vi "final_usrp_transceiver_webcam.vi"() -> ()   [LabVIEW 2014]
uses:
  <vilib>/userdefined/High Color/IMAQdx.ctl
  <vilib>/addons/Modulation/Analog/support/mod_Set Error Source.vi
  var_stop.vi
  <vilib>/addons/Modulation/Digital/Support/Common/Validators/mod_Generate Filter Coefficients Validate.vi
  <vilib>/addons/Modulation/Digital/General/subVIs/mod_Generate Filter Coefficients.vi
  <vilib>/measure/maspectr.llb/FFT Power Spectrum and PSD for 1 Chan (CDB).vi
  <vilib>/addons/Modulation/Digital/General/MT Apply Matched Filter (Generic).vi
  <vilib>/addons/Modulation/Digital/General/MT Align to Ideal Symbols (Generic).vi
  <instrlib>/niUSRP/niUSRP Fetch Rx Data (CDB Cluster).vi
  <instrlib>/niUSRP/niUSRP Write Tx Data (CDB Cluster).vi
  <vilib>/addons/Modulation/Digital/General/MT Apply Pulse Shaping Filter (Generic).vi
  <vilib>/addons/Modulation/niDMT.lvlib
  <vilib>/measure/NI_MAPro.lvlib
  <vilib>/vision/driver/NI_Vision_Acquisition_Software.lvlib
panel:
  out "RX Constellation Map 2":cdb[](graph)
  in  "Modulation 2":enum16{"PSK", "QAM"}(ring)=enum."QAM"
  out "error out":errorcluster
  in  "cam":T1
  in  "frame buffer size":i32=20
  in  "Stop":bool
  in  "energy threshold":dbl=-33.0 format="%#_13g"
  out "elements in frame buffer 2":i32
  out "elements in frame buffer":i32
  out "valid frames":i32
  out "elements in send buffer":i32
  in  "packet size":i32=12800
  in  "Quality (0-1000)":i32=100 caption="Quality (750)"
  out "size(s) 4":i32
  out "frame num":u32
  out "length":i32[](array[numeric])
  out "start index":i32[](array[numeric])
  out "Numeric":i32
  out "size(s) 3":i32
  out "# elements in queue 2":i32
  out "size(s) 2":i32
  out "size(s)":i32[](array[numeric])
  out "image":T2(plugin-control)
  in  "Transmit power (db)":dbl
  out "found?":bool
  out "# elements in queue":i32
  out "valid?":bool
  in  "Gray code?":bool=TRUE
  in  "Modulation":enum16{"PSK", "QAM"}(ring)
  out "packet len":u32
  in  "filter length (symbols)":i32=8
  in  "filter parameter":dbl=0.5 format="%.2f"
  in  "pulse shaping filter (none)":T3(ring)=enum."Raised Cosine"
  in  "M-PSK (4)":i32=4 caption="M-ARY"
  in  "samples per symbol (16)":i32=4
  out "packet bits length":i32
  in  "number of samples":i64=40000
  out "RX coerced gain":dbl format="%#_6f"
  out "RX coerced carrier frequency":dbl=915000000.0 format="%#_6p"
  out "RX coerced IQ rate":dbl=4000000.0 format="%#_6p"
  in  "RX active antenna":string="RX2"
  in  "RX gain":dbl format="%#_6f"
  in  "RX device names":refnum<k15>="192.168.10.2"
  out "TX coerced gain":dbl format="%#_6f"
  out "TX coerced carrier frequency":dbl=915000000.0 format="%#_6p"
  out "coerced IQ rate":dbl=4000000.0 format="%#_6p"
  in  "TX device names":refnum<k15>="192.168.10.2"
  in  "TX gain":dbl format="%#_6f"
  in  "carrier frequency":dbl=915000000.0 format="%#_6p"
  in  "IQ rate":dbl=800000.0 format="%#_6p"
  in  "stop":bool
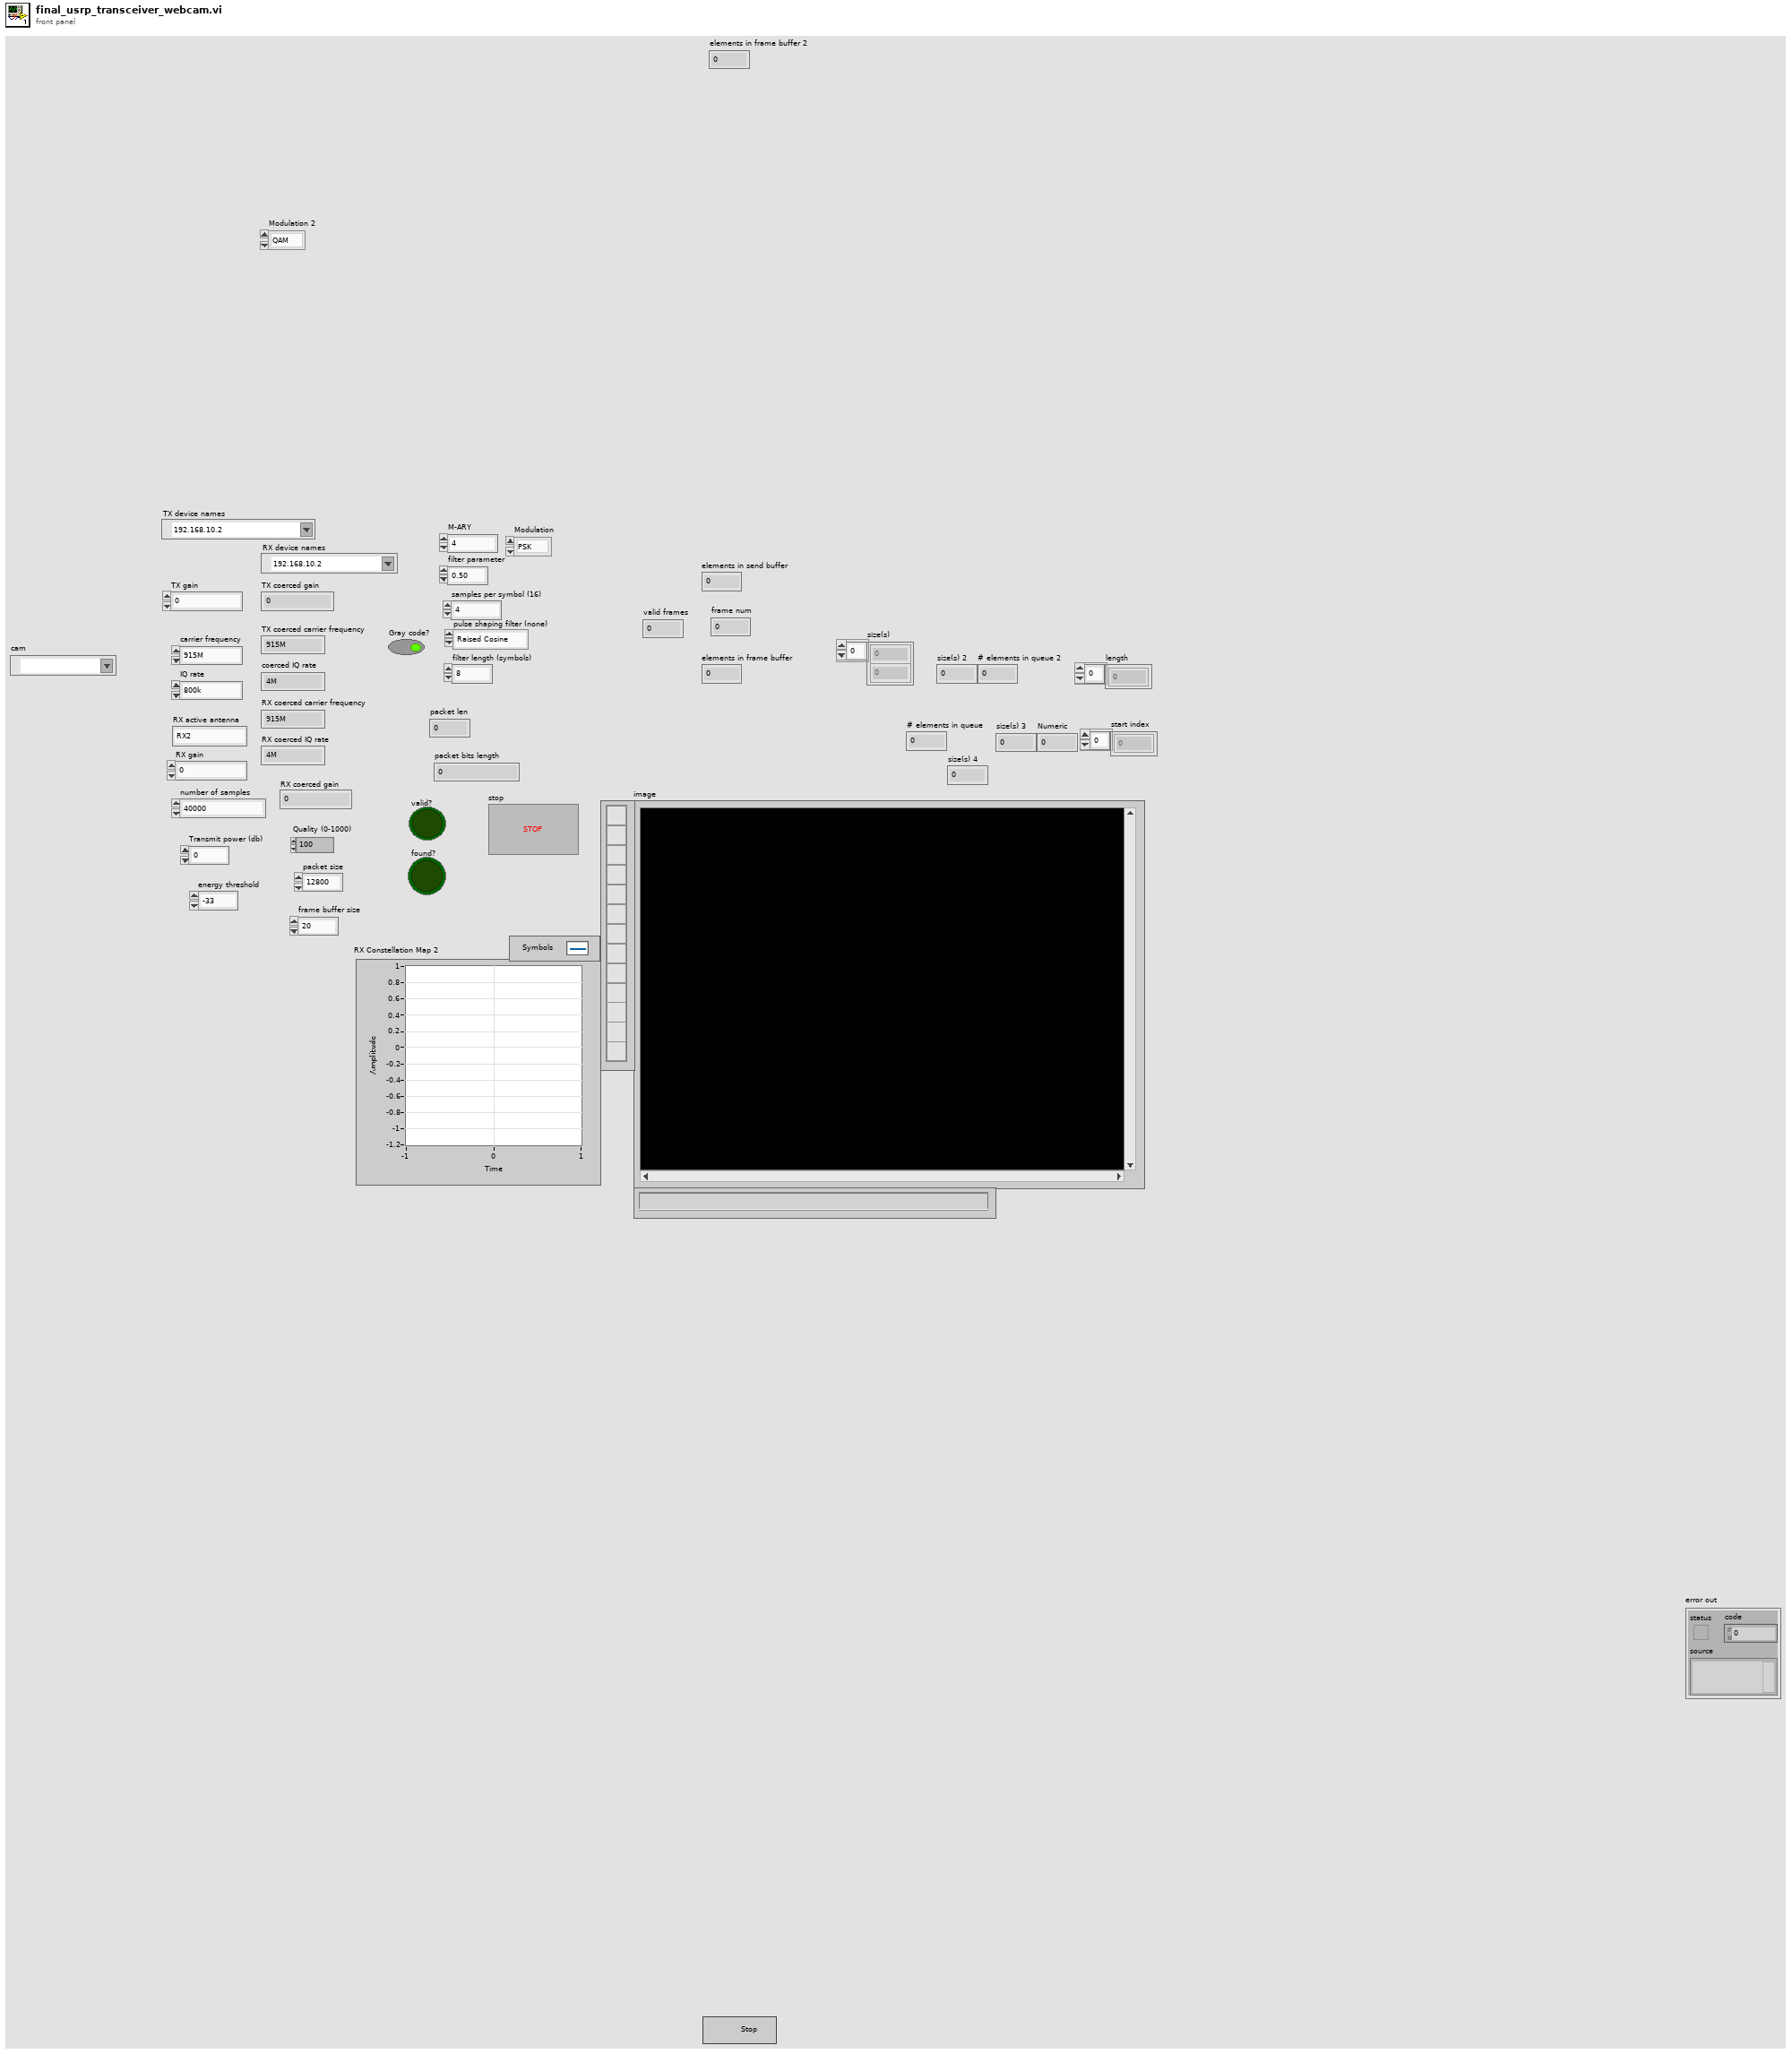
[diagram p1: front panel]
types:
  T1 = typedef "IMAQdx.ctl" = refnum<k21>
  T2 = typedef "IMAQ Image.ctl" = refnum<image>
  T3 = enum16{"none", "Raised Cosine", "Root Raised Cos", "Gaussian"}
  T4 = typedef "Image Type" = u32
  T5 = enum16{"FSK", "PSK", "QAM", "MSK", "PAM", "ASK", "CPM"}
  T6 = cluster{"samples per symbol (16)":i32, "symbol map":cdb[], "index map":u32[]}
  T7 = cluster{"samples per symbol (16)":i32, "symbol map":cdb[], i32[]}
  T8 = typedef "Semaphore RefNum" = refnum<k1>
  T9 = typedef "niAMT.lvlib/Complex Data Waveform.ctl" = cluster{"t0":dbl, "dt":dbl, "Y":cdb[]}
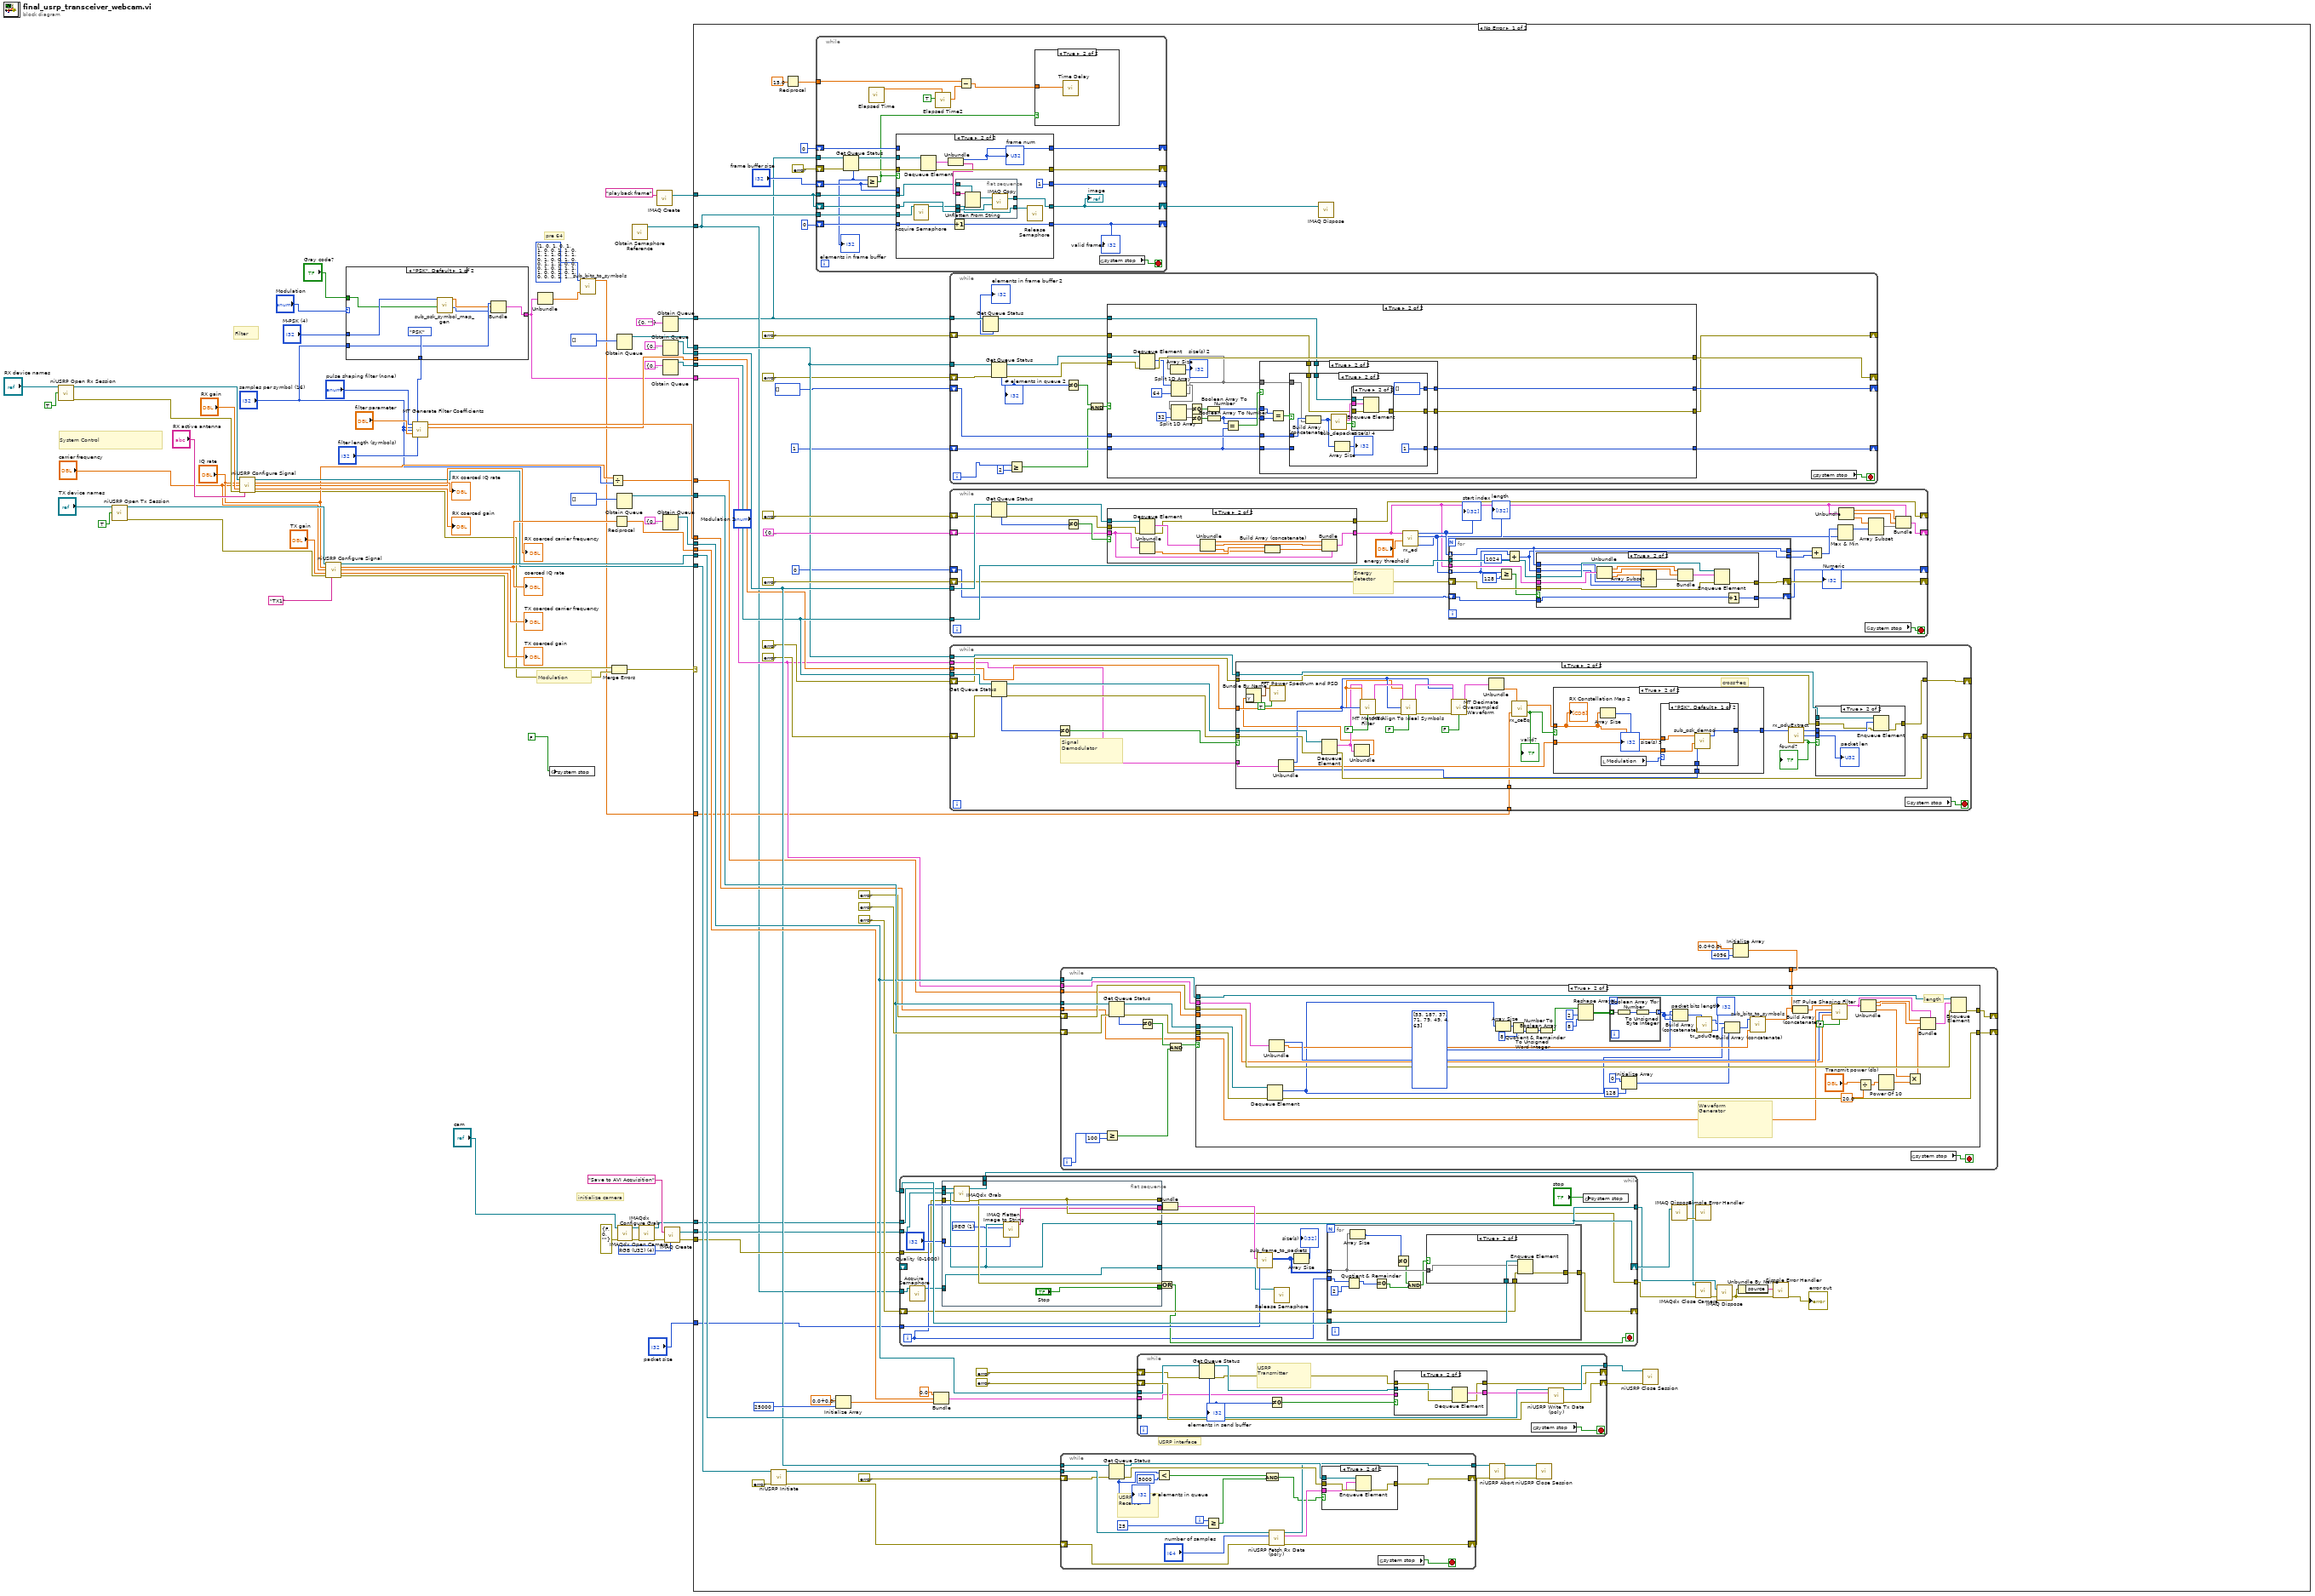
[diagram p0: block diagram]
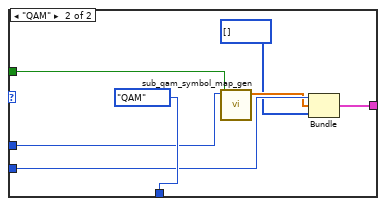
[diagram p2: hidden frame]
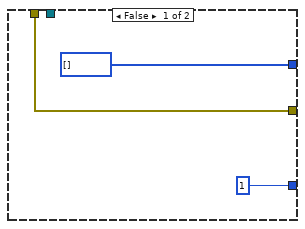
[diagram p7: hidden frame]
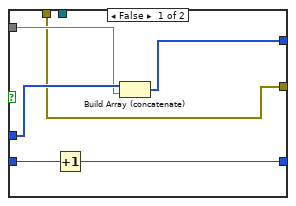
[diagram p8: hidden frame]
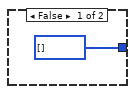
[diagram p11: hidden frame]
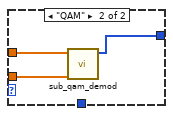
[diagram p12: hidden frame]
diagram:
  w11 = T4 4 items=["Grayscale (U8)", "Grayscale (I16)", "Grayscale (SGL)", "Complex (CSG)", "RGB (U32)", "HSL (U32)", "RGB (U64)", "Grayscale (U16)"] ("Image Type")
  # "initialize camera"
  # "pre 64"
  # "Modulation"
  # "Filter"
  # "System Control"
  n1 = call <instrlib>:"niUSRP Open Rx Session.vi"("device names"="RX device names", "reset"=TRUE) -> ("session handle out"=w54:refnum<k15>, "error out"=w53:errorcluster)  [unwired: 12 in]
  n2 = call <instrlib>:"niUSRP Open Tx Session.vi"("device names"="TX device names", "reset"=TRUE) -> ("session handle out"=w67:refnum<k15>, "error out"=w66:errorcluster)  [unwired: 12 in]
  n3 = call <instrlib>:"niUSRP Configure Signal.vi"("session handle"=w54, "IQ rate"="IQ rate", "carrier frequency"="carrier frequency", "gain"="RX gain", "error in (no error)"=w53, "active antenna"="RX active antenna") -> ("session handle out"=w45:refnum<k15>, "coerced IQ rate"=→"RX coerced IQ rate":dbl, "coerced carrier frequency"=→"RX coerced carrier frequency":dbl, "coerced gain"=→"RX coerced gain":dbl, "error out"=w29:errorcluster)  [unwired: 5 in]
  n4 = call <instrlib>:"niUSRP Configure Signal.vi"("session handle"=w67, "IQ rate"="IQ rate", "carrier frequency"="carrier frequency", "gain"="TX gain", "error in (no error)"=w66, "active antenna"="TX1") -> ("session handle out"=w58:refnum<k15>, "coerced IQ rate"=w56:dbl, "coerced carrier frequency"=→"TX coerced carrier frequency":dbl, "coerced gain"=→"TX coerced gain":dbl, "error out"=w30:errorcluster)  [unwired: 5 in]
  "coerced IQ rate" <- w56
  n5 = case shown="\"PSK\", Default" "Modulation" {
    tunnel: [T5."PSK" ("modulation type") T5."QAM" ("modulation type")] -> w24
    tunnel: "M-PSK (4)" -> [w74 w80]
    tunnel: "Gray code?" -> [w73 w81]
    tunnel: "samples per symbol (16)" -> [w72 w79]
    tunnel: [w69 w76] -> w17
    frame "PSK", Default {
      n6 = call "sub_psk_symbol_map_gen.vi"("Gray code?"=w73, "M-PSK"=w74) -> ("index map"=w70:u32[], "symbol map"=w71:cdb[])  [unwired: 8 in]
      n7 = Bundle("samples per symbol (16)"=w72, "symbol map"=w71, "index map"=w70) -> (w69:T6)  [unwired: 1 in]
    }
    frame "QAM" {
      n8 = call "sub_qam_symbol_map_gen.vi"("Gray code?"=w81, "M-QAM"=w80) -> ("symbol map"=w78:cdb[])  [unwired: 9 in]
      n9 = Bundle("samples per symbol (16)"=w79, "symbol map"=w78, i32[] []) -> (w76:T7)  [unwired: 1 in]
    }
  }
  n10 = call <vilib>:"MT Generate Filter Coefficients.vi"("pulse shaping filter (none)"="pulse shaping filter (none)", "modulation type"=w24, "pulse shaping samples per symbol (16)"="samples per symbol (16)", "matched samples per symbol (16)"="samples per symbol (16)", "filter parameter"="filter parameter", "filter length (symbols)"="filter length (symbols)") -> ("pulse shaping filter coefficients"=w35:dbl[], "matched filter coefficients"=w33:dbl[])  [unwired: 7 in, 1 out]
  n11 = Unbundle(w17) -> ("symbol map"=w19:cdb[])  [unwired: 2 out]
  n12 = global write "var_stop.vi" "system stop"(FALSE) -> ()
  n13 = call "sub_bits_to_symbols.vi"("symbol map"=w19, "bits"=i16[] [1, 0, 1, 0, 1, 1, 0, 0, 1, 1, 0, 1, 1, 1, 0, 1, 1, 0, 1, 0, 0, 1, 0, 0, 1, 1, 1, 0, 0, 0, 1, 0, 1, 1, 1, 1, 0, 0, 1, 0, 1, 0, 0, 0, 1, 1, 0, 0, 0, 0, 1, 0, 0, 0, 0, 0, 1, 1, 1, 1, 1, 1, 0, 0] ("preamble(64) 2")) -> ("symbols"=w18:cdb[])  [unwired: 9 in]
  n14 = Divide(x="IQ rate", y="samples per symbol (16)") -> (x/y=w34:dbl)
  n15 = Merge Errors(w30, w29) -> (w28:errorcluster)
  n16 = Reciprocal(x=w56) -> (1/x=w55:dbl)
  n17 = Obtain Queue(element data type=i8[] [] ("output bit stream")) -> (queue out=w40:refnum<queue>)  [unwired: 4 in, 2 out]
  n18 = Obtain Queue(element data type=i16[] []) -> (queue out=w68:refnum<queue>)  [unwired: 4 in, 2 out]
  n19 = call <vilib>:"IMAQdx Open Camera.vi"("error in"=errorcluster {"status"=FALSE, "code"=0, "source"=""}, "Session In"="cam") -> ("error out"=w7:errorcluster, "Session Out"=w9:T1)  [unwired: 8 in]
  n20 = call <vilib>:"Obtain Semaphore Reference.vi"() -> ("semaphore"=w1:T8)  [unwired: 5 in, 2 out]
  n21 = call <vilib>:"IMAQdx Configure Grab.vi"("error in"=w7, "Session In"=w9) -> ("error out"=w6:errorcluster, "Session Out"=w4:T1)  [unwired: 8 in]
  n22 = call "IMAQ Create"("Image Name"="playback frame") -> ("New Image"=w12:T2)  [unwired: 3 in, 2 out]
  n23 = Obtain Queue(element data type=cluster{u32, "string":string} {0, "string"=""} ("frame")) -> (queue out=w15:refnum<queue>)  [unwired: 4 in, 2 out]
  n24 = Obtain Queue(element data type=cluster{"t0":dbl, "dt":dbl, "Y":cdb[]} {"t0"=0.0, "dt"=0.0, "Y"=[]} ("data")) -> (queue out=w44:refnum<queue>)  [unwired: 4 in, 2 out]
  n25 = Obtain Queue(element data type=cluster{"t0":dbl, "dt":dbl, "Y":cdb[]} {"t0"=0.0, "dt"=0.0, "Y"=[]} ("data")) -> (queue out=w41:refnum<queue>)  [unwired: 4 in, 2 out]
  n26 = Obtain Queue(element data type=cluster{"t0":dbl, "dt":dbl, "Y":cdb[]} {"t0"=0.0, "dt"=1.0, "Y"=[]} ("data")) -> (queue out=w59:refnum<queue>)  [unwired: 4 in, 2 out]
  n27 = call "IMAQ Create"("Image Name"="Save to AVI Acquisition", "Image Type"=w11, "error in (no error)"=w6) -> ("New Image"=w5:T2, "error out"=w3:errorcluster)  [unwired: 2 in]
  n28 = case shown="No Error" w28 {
    tunnel: w68 -> [w150 _]
    tunnel: w59 -> [w145 _]
    tunnel: w58 -> [w146 _]
    tunnel: w55 -> [w139 _]
    tunnel: w45 -> [w134 _]
    tunnel: w44 -> [w128 _]
    tunnel: w41 -> [w124 _]
    tunnel: w40 -> [w122 _]
    tunnel: w17 -> [w116 _]
    tunnel: w35 -> [w119 _]
    tunnel: w34 -> [w118 _]
    tunnel: w33 -> [w117 _]
    tunnel: w18 -> [w110 _]
    tunnel: w15 -> [w83 _]
    tunnel: "packet size" -> [w101 _]
    tunnel: w12 -> [w95 _]
    tunnel: w5 -> [w94 _]
    tunnel: w4 -> [w93 _]
    tunnel: w3 -> [w92 _]
    tunnel: w1 -> [w84 _]
    frame No Error {
      # "USRP interface"
      n29 = call <instrlib>:"niUSRP Initiate.vi"("session handle"=w134, "error in (no error)"=errorcluster {"status"=FALSE, "code"=0, "source"=""}) -> ("session handle out"=w133:refnum<k15>, "error out"=w132:errorcluster)  [unwired: 12 in]
      n30 = Reciprocal(x=15.0) -> (1/x=w102:dbl)
      n31 = while {
        tunnel: w83 -> [w223]
        shift-right: [w219] -> _
        shift-left: errorcluster {"status"=FALSE, "code"=0, "source"=""} ("error out") -> [w222]
        shift-right: [w216] -> _
        shift-left: 0 -> [w215]
        tunnel: w102 -> [w211]
        shift-right: [w212] -> _
        shift-left: 0 -> [w213]
        shift-right: [w208] -> _
        shift-left: "frame buffer size" -> [w207]
        shift-right: [w204] -> w96
        shift-left: w95 -> [w205]
        tunnel: w95 -> [w203]
        tunnel: w84 -> [w202]
        stop <- w218 stop-if-true
        n32 = Get Queue Status(queue=w223, error in (no error)=w222) -> (queue out=w221:refnum<queue>, error out=w220:errorcluster, # elements in queue=w201:i32)  [unwired: 1 in, 5 out]
        "elements in frame buffer" <- w201
        n33 = Greater Or Equal?(x=w201, y=w207) -> (x >= y?=w206:bool)
        n34 = call "Elapsed Time"() -> ("Present (s)"=w210:dbl)  [unwired: 12 in, 7 out]
        n35 = case shown="True" w206 {
          tunnel: w221 -> [_ w244]
          tunnel: w220 -> [w229 w243]
          tunnel: [w229 w241] -> w219
          tunnel: [w228 w240] -> w216
          tunnel: w215 -> [w228 _]
          tunnel: w213 -> [w227 w239]
          tunnel: [w227 w238] -> w212
          tunnel: [w226 1] -> w208
          tunnel: w207 -> [w226 _]
          tunnel: [w225 w230] -> w204
          tunnel: w205 -> [w225 w233]
          tunnel: w203 -> [_ w234]
          tunnel: w202 -> [_ w236]
          frame False {
          }
          frame True {
            n36 = call <vilib>:"Acquire Semaphore.vi"("semaphore"=w236) -> ("semaphore out"=w232:T8)  [unwired: 4 in, 2 out]
            n37 = Dequeue Element(queue=w244, error in (no error)=w243) -> (element=w242:cluster{u32, "string":string}, error out=w241:errorcluster)  [unwired: 1 in, 2 out]
            n38 = Unbundle(w242) -> (w240:u32, "string"=w235:string)
            "frame num" <- w240
            n39 = Increment(x=w239) -> (x+1=w238:i32)
            n40 = flat-sequence {
              tunnel: w235 -> [w250]
              tunnel: w234 -> [w249]
              tunnel: [w247] -> w230
              tunnel: w233 -> [w246]
              tunnel: w232 -> [w245]
              tunnel: [w245] -> w231
              frame #0 {
                n41 = Unflatten From String(type=w249, binary string=w250) -> (value=w248:T2)  [unwired: 3 in, 2 out]
                n42 = call "IMAQ Copy"("Image Dst"=w246, "Image Src"=w248) -> ("Image Dst Out"=w247:T2)  [unwired: 4 in, 1 out]
              }
            }
            n43 = call <vilib>:"Release Semaphore.vi"("semaphore"=w231) -> ()  [unwired: 5 in, 2 out]
          }
        }
        "valid frames" <- w212
        "image" <- w204
        n44 = call "Elapsed Time2"("Reset"=TRUE, "Set Start Time (s)"=w210) -> ("Elapsed Time (s)"=w214:dbl)  [unwired: 10 in, 7 out]
        n45 = Subtract(x=w211, y=w214) -> (x-y=w209:dbl)
        n46 = case shown="True" w206 {
          tunnel: w209 -> [_ w224]
          frame False {
          }
          frame True {
            n47 = call "Time Delay"("Delay Time (s)"=w224) -> ()  [unwired: 10 in, 1 out]
          }
        }
        n48 = global read "var_stop.vi" "system stop"() -> (w218:bool)
      }
      n49 = Initialize Array(cdb 0.0+0.0i, 25000 ("dimension size")) -> (w140:cdb[])
      n50 = while {
        tunnel: w150 -> [w172]
        shift-right: [w170] -> _
        shift-left: errorcluster {"status"=FALSE, "code"=0, "source"=""} ("error out") -> [w171]
        tunnel: w101 -> [w167]
        tunnel: [w162] -> w87
        shift-right: [w162] -> w97
        shift-left: _ -> [_]
        tunnel: w92 -> [w159]
        tunnel: w94 -> [w160]
        tunnel: w93 -> [w161]
        tunnel: [w158] -> w86
        tunnel: [w157] -> w85
        tunnel: w84 -> [w156]
        i -> [w163]
        stop <- w164 stop-if-true
        n51 = call <vilib>:"Acquire Semaphore.vi"("semaphore"=w156) -> ("semaphore out"=w153:T8)  [unwired: 4 in, 2 out]
        n52 = flat-sequence {
          tunnel: "Quality (0-1000)" -> [w184]
          tunnel: [w183] -> w162
          tunnel: w161 -> [w182]
          tunnel: w160 -> [w181]
          tunnel: w159 -> [w180]
          tunnel: [w179] -> w158
          tunnel: [w178] -> w157
          tunnel: ["Stop"] -> w155
          tunnel: [w175] -> w154
          tunnel: [w174] -> _
          tunnel: w153 -> [w174]
          tunnel: [w174] -> w152
          frame #0 {
            w176 = 1 items=["None", "JPEG", "PACKED BINARY"] ("Compression (None)")
            n53 = call <vilib>:"IMAQdx Grab.vi"("error in"=w180, "Image In"=w181, "Session In"=w182) -> ("error out"=w178:errorcluster, "Image Out"=w183:T2, "Session Out"=w179:T1)  [unwired: 5 in, 1 out]
            n54 = call "IMAQ Flatten Image to String"("Quality (750)"=w184, "Compression (None)"=w176, "Image"=w183) -> ("Data String"=w175:string)  [unwired: 7 in, 1 out]
          }
        }
        n55 = Or(x=w157, y=w155) -> (x .or. y?=w164:bool)
        n56 = Bundle(w163, "Data String"=w154) -> (w166:cluster{i32, "Data String":string})  [unwired: 1 in]
        n57 = call "sub_frame_to_packets.vi"("packet size"=w167, "Cluster"=w166) -> ("packets"=w169:i16[][])  [unwired: 9 in]
        n58 = call <vilib>:"Release Semaphore.vi"("semaphore"=w152) -> ()  [unwired: 5 in, 2 out]
        n59 = Array Size(array=w169) -> (size(s)=→"size(s)":i32[])
        n60 = for {
          tunnel: w172 -> [w195]
          tunnel: w171 -> [w194]
          tunnel: [w193] -> w170
          tunnel: w169 -> [w191] mode=indexing
          tunnel: w163 -> [w190]
          n61 = Quotient & Remainder(x=w190, y=2) -> (x-y*floor(x/y)=w188:i32)  [unwired: 1 out]
          n62 = Array Size(array=w191) -> (size(s)=w192:i32)
          n63 = Equal To 0?(x=w188) -> (x = 0?=w187:bool)
          n64 = Not Equal To 0?(x=w192) -> (x != 0?=w186:bool)
          n65 = And(x=w186, y=w187) -> (x .and. y?=w185:bool)
          n66 = case shown="True" w185 {
            tunnel: w191 -> [_ w197]
            tunnel: w195 -> [_ w200]
            tunnel: w194 -> [w196 w199]
            tunnel: [w196 w198] -> w193
            frame False {
            }
            frame True {
              n67 = Enqueue Element(queue=w200, element=w197, error in (no error)=w199) -> (error out=w198:errorcluster)  [unwired: 1 in, 2 out]
            }
          }
        }
        n68 = global write "var_stop.vi" "system stop"("stop") -> ()
      }
      n69 = Bundle(0.0, w139, w140) -> (w137:cluster{dbl, dbl, cdb[]})  [unwired: 1 in]
      n70 = while {
        tunnel: w122 -> [w271]
        shift-right: [w264] -> _
        shift-left: errorcluster {"status"=FALSE, "code"=0, "source"=""} ("error out") -> [w270]
        shift-right: [w262] -> _
        shift-left: u32 1 -> [w263]
        shift-right: [w261] -> _
        shift-left: i8[] [] ("second subarray") -> [w260]
        tunnel: w83 -> [w259]
        shift-right: [w257] -> _
        shift-left: errorcluster {"status"=FALSE, "code"=0, "source"=""} ("error out") -> [w258]
        i -> [w255]
        stop <- w269 stop-if-true
        n71 = Get Queue Status(queue=w259) -> (queue out=w252:refnum<queue>, # elements in queue=→"elements in frame buffer 2":i32)  [unwired: 2 in, 6 out]
        n72 = Get Queue Status(queue=w271, error in (no error)=w270) -> (queue out=w266:refnum<queue>, error out=w265:errorcluster, # elements in queue=w268:i32)  [unwired: 1 in, 5 out]
        "# elements in queue 2" <- w268
        n73 = Greater Or Equal?(x=w255, y=2) -> (x >= y?=w254:bool)
        n74 = Not Equal To 0?(x=w268) -> (x != 0?=w267:bool)
        n75 = And(x=w267, y=w254) -> (x .and. y?=w253:bool)
        n76 = case shown="True" w253 {
          tunnel: w266 -> [_ w298]
          tunnel: w265 -> [w275 w297]
          tunnel: [w275 w296] -> w264
          tunnel: w263 -> [w274 w282]
          tunnel: [w274 w283] -> w262
          tunnel: [w272 w287] -> w261
          tunnel: w260 -> [w272 w284]
          tunnel: w252 -> [_ w281]
          tunnel: w258 -> [w273 w280]
          tunnel: [w273 w279] -> w257
          frame False {
          }
          frame True {
            n77 = Dequeue Element(queue=w298, error in (no error)=w297) -> (element=w278:i8[], error out=w296:errorcluster)  [unwired: 1 in, 2 out]
            n78 = Split 1D Array(array=w278, index=64) -> (first subarray=w289:i8[], second subarray=w276:i8[])
            n79 = Array Size(array=w276) -> (size(s)=→"size(s) 2":i32)
            n80 = Split 1D Array(array=w289, index=32) -> (first subarray=w292:i8[], second subarray=w293:i8[])
            n81 = Not Equal To 0?(x=w292) -> (x != 0?=w291:bool[])
            n82 = Not Equal To 0?(x=w293) -> (x != 0?=w290:bool[])
            n83 = Boolean Array To Number(Boolean array=w291) -> (number=w286:u32)
            n84 = Boolean Array To Number(Boolean array=w290) -> (number=w285:u32)
            n85 = Equal?(x=w285, y=w282) -> (x = y?=w288:bool)
            n86 = case shown="True" w288 {
              tunnel: [i8[] [] ("second subarray") w309] -> w287
              tunnel: w286 -> [_ w312]
              tunnel: w285 -> [_ w311]
              tunnel: w284 -> [_ w308]
              tunnel: w276 -> [_ w307]
              tunnel: [u32 1 w306] -> w283
              tunnel: w282 -> [_ w305]
              tunnel: w281 -> [_ w304]
              tunnel: w280 -> [w299 w303]
              tunnel: [w299 w302] -> w279
              frame False {
              }
              frame True {
                n87 = Equal?(x=w312, y=w311) -> (x = y?=w310:bool)
                n88 = case shown="True" w310 {
                  tunnel: [w316 i8[] [] ("second subarray")] -> w309
                  tunnel: w308 -> [w318 w327]
                  tunnel: w307 -> [w317 w326]
                  tunnel: [w314 u32 1] -> w306
                  tunnel: w305 -> [w315 _]
                  tunnel: w304 -> [_ w325]
                  tunnel: w303 -> [w313 w323]
                  tunnel: [w313 w322] -> w302
                  frame False {
                    n89 = Increment(x=w315) -> (x+1=w314:u32)
                    n90 = Build Array (concatenate)(w318, w317) -> (w316:i8[])
                  }
                  frame True {
                    n91 = Build Array (concatenate)(w327, w326) -> (w321:i8[])
                    n92 = call "sub_depacket.vi"("bitstream"=w321) -> ("CRC valid"=w319:bool, "frame"=w324:cluster{u32, "string":string})  [unwired: 9 in]
                    n93 = Array Size(array=w321) -> (size(s)=→"size(s) 4":i32)
                    n94 = case shown="True" w319 {
                      tunnel: w325 -> [_ w334]
                      tunnel: w324 -> [_ w333]
                      tunnel: w323 -> [w330 w332]
                      tunnel: [w330 w331] -> w322
                      frame False {
                      }
                      frame True {
                        n95 = Enqueue Element(queue=w334, element=w333, error in (no error)=w332) -> (error out=w331:errorcluster)  [unwired: 1 in, 2 out]
                      }
                    }
                  }
                }
              }
            }
          }
        }
        n96 = global read "var_stop.vi" "system stop"() -> (w269:bool)
      }
      n97 = while {
        tunnel: w128 -> [w429]
        shift-right: [w422] -> _
        shift-left: errorcluster {"status"=FALSE, "code"=0, "source"=""} ("error out") -> [w428]
        shift-right: [w408] -> _
        shift-left: cluster{"t0":dbl, "dt":dbl, "Y":cdb[]} {"t0"=0.0, "dt"=0.0, "Y"=[]} ("data") -> [w423]
        tunnel: w124 -> [w421]
        shift-right: [w420] -> _
        shift-left: errorcluster {"status"=FALSE, "code"=0, "source"=""} ("error out") -> [w419]
        shift-right: [w403] -> _
        shift-left: 0 -> [w404]
        stop <- w418 stop-if-true
        # "Energy\ndetector"
        n98 = Get Queue Status(queue=w429, error in (no error)=w428) -> (queue out=w424:refnum<queue>, error out=w425:errorcluster, # elements in queue=w427:i32)  [unwired: 1 in, 5 out]
        n99 = Not Equal To 0?(x=w427) -> (x != 0?=w426:bool)
        n100 = case shown="True" w426 {
          tunnel: w425 -> [w458 w469]
          tunnel: w424 -> [_ w468]
          tunnel: w423 -> [w457 w463]
          tunnel: [w458 w460] -> w422
          tunnel: [w457 w459] -> w415
          frame False {
          }
          frame True {
            n101 = Unbundle(w463) -> ("Y"=w466:cdb[])  [unwired: 2 out]
            n102 = Dequeue Element(queue=w468, error in (no error)=w469) -> (element=w467:cluster{"t0":dbl, "dt":dbl, "Y":cdb[]}, error out=w460:errorcluster)  [unwired: 1 in, 2 out]
            n103 = Unbundle(w467) -> ("t0"=w462:dbl, "dt"=w461:dbl, "Y"=w465:cdb[])
            n104 = Build Array (concatenate)(w466, w465) -> (w464:cdb[])
            n105 = Bundle(cluster=w463, "t0"=w462, "dt"=w461, "Y"=w464) -> (w459:cluster{"t0":dbl, "dt":dbl, "Y":cdb[]})
          }
        }
        n106 = call "rx_ed.vi"("energy threshold"="energy threshold", "Wavefrom"=w415) -> ("first pulse"=w405:i32, "length"=w416:i32[], "start index"=w417:i32[])  [unwired: 7 in]
        "start index" <- w417
        "length" <- w416
        n107 = for {
          tunnel: w421 -> [w441]
          tunnel: w415 -> [w438]
          shift-right: [w440] -> w420
          shift-left: w419 -> [w439]
          tunnel: w417 -> [w437] mode=indexing
          tunnel: w416 -> [w432] mode=indexing
          tunnel: [w437] -> w411
          tunnel: [w430] -> w410
          shift-right: [w433] -> w403
          shift-left: w404 -> [w434]
          n108 = Greater Or Equal?(x=w432, y=128) -> (x >= y?=w435:bool)
          n109 = Add(x=w432, y=1024) -> (x+y=w430:i32)
          n110 = case shown="True" w435 {
            tunnel: w441 -> [_ w456]
            tunnel: [w443 w455] -> w440
            tunnel: w439 -> [w443 w454]
            tunnel: w438 -> [_ w453]
            tunnel: w437 -> [_ w447]
            tunnel: w430 -> [_ w446]
            tunnel: w434 -> [w442 w445]
            tunnel: [w442 w444] -> w433
            frame False {
            }
            frame True {
              n111 = Unbundle(w453) -> ("t0"=w451:dbl, "dt"=w452:dbl, "Y"=w449:cdb[])
              n112 = Array Subset(array=w449, index=w447, length=w446) -> (w448:cdb[])
              n113 = Bundle("t0"=w451, "dt"=w452, w448) -> (w450:cluster{"t0":dbl, "dt":dbl, cdb[]})  [unwired: 1 in]
              n114 = Enqueue Element(queue=w456, element=w450, error in (no error)=w454) -> (error out=w455:errorcluster)  [unwired: 1 in, 2 out]
              n115 = Increment(x=w445) -> (x+1=w444:i32)
            }
          }
        }
        "Numeric" <- w403
        n116 = Add(x=w411, y=w410) -> (x+y=w407:i32)
        n117 = Max & Min(x=w407, y=w405) -> (max(x,y)=w406:i32)  [unwired: 1 out]
        n118 = Unbundle(w415) -> ("t0"=w414:dbl, "dt"=w413:dbl, "Y"=w412:cdb[])
        n119 = global read "var_stop.vi" "system stop"() -> (w418:bool)
        n120 = Array Subset(array=w412, index=w406) -> (w409:cdb[])  [unwired: 1 in]
        n121 = Bundle(cluster=w415, "t0"=w414, "dt"=w413, "Y"=w409) -> (w408:cluster{"t0":dbl, "dt":dbl, "Y":cdb[]})
      }
      n122 = while {
        tunnel: w124 -> [w348]
        shift-right: [w342] -> _
        shift-left: errorcluster {"status"=FALSE, "code"=0, "source"=""} ("error out") -> [w347]
        tunnel: w122 -> [w341]
        shift-right: [w340] -> _
        shift-left: errorcluster {"status"=FALSE, "code"=0, "source"=""} ("error out") -> [w339]
        tunnel: w117 -> [w337]
        tunnel: w116 -> [w336]
        tunnel: w110 -> [w335]
        stop <- w338 stop-if-true
        # "Signal \nDemodulator"
        n123 = Get Queue Status(queue=w348, error in (no error)=w347) -> (queue out=w344:refnum<queue>, error out=w343:errorcluster, # elements in queue=w346:i32)  [unwired: 1 in, 5 out]
        n124 = Not Equal To 0?(x=w346) -> (x != 0?=w345:bool)
        n125 = case shown="True" w345 {
          tunnel: w344 -> [_ w380]
          tunnel: w343 -> [w350 w381]
          tunnel: [w350 w379] -> w342
          tunnel: w341 -> [_ w370]
          tunnel: [w349 w369] -> w340
          tunnel: w339 -> [w349 w368]
          tunnel: w337 -> [_ w357]
          tunnel: w336 -> [_ w361]
          tunnel: w335 -> [_ w354]
          frame False {
          }
          frame True {
            # "cross+eq"
            n126 = Unbundle(w361) -> ("samples per symbol (16)"=w360:i32, "symbol map"=w359:cdb[], "index map"=w358:u32[])
            n127 = Dequeue Element(queue=w380, error in (no error)=w381) -> (element=w353:cluster{"t0":dbl, "dt":dbl, "Y":cdb[]}, error out=w379:errorcluster)  [unwired: 1 in, 2 out]
            n128 = Unbundle(w353) -> ("Y"=w352:cdb[])  [unwired: 2 out]
            n129 = Bundle By Name("Y"=w352) -> (w356:waveform(cdb))  [unwired: 1 in]
            n130 = call-poly <vilib>:"FFT Power Spectrum and PSD.vi"("dB On (F)"=TRUE, "time signal"=w356) -> ()  [unwired: 6 in, 4 out]
            n131 = call-poly <vilib>:"MT Matched Filter.vi"("input complex waveform"=w353, "matched filter coefficients"=w357, "samples per symbol (16)"=w360, "reset? (T)"=FALSE) -> ("output complex waveform"=w378:T9, "error out"=w377:errorcluster)  [unwired: 10 in]
            n132 = call-poly <vilib>:"MT Align To Ideal Symbols.vi"("input complex waveform"=w378, "matched filter coefficients"=w357, "samples per symbol (16)"=w360, "error in (no error)"=w377, "reset? (T)"=FALSE) -> ("output complex waveform"=w375:T9, "error out"=w376:errorcluster)  [unwired: 8 in, 1 out]
            n133 = call <vilib>:"MT Decimate Oversampled Waveform.vi"("input complex waveform"=w375, "decimation factor"=w360, "error in (no error)"=w376, "reset? (T)"=FALSE) -> ("output complex waveform"=w351:T9)  [unwired: 10 in, 1 out]
            n134 = Unbundle(w351) -> ("Y"=w371:cdb[])  [unwired: 2 out]
            n135 = call "rx_ceEq.vi"("preamble"=w354, "symbols"=w371) -> ("valid?"=w366:bool, "eq symbols"=w367:cdb[])
            "valid?" <- w366
            n136 = case shown="True" w366 {
              tunnel: [i8[] [] ("output bit stream") w386] -> w374
              tunnel: w359 -> [_ w387]
              tunnel: w367 -> [_ w383]
              tunnel: w358 -> [_ w385]
              frame False {
              }
              frame True {
                n137 = Array Size(array=w383) -> (size(s)=→"size(s) 3":i32)
                n138 = local read "Modulation"() -> (w388:enum16{"PSK", "QAM"})
                n139 = case shown="\"PSK\", Default" w388 {
                  tunnel: w383 -> [w392 w395]
                  tunnel: w387 -> [w391 w394]
                  tunnel: [w389 w393] -> w386
                  tunnel: w385 -> [w390 _]
                  frame "PSK", Default {
                    n140 = call "sub_psk_demod.vi"("index map"=w390, "symbol map"=w391, "symbol"=w392) -> ("bitstream"=w389:i16[])  [unwired: 8 in]
                  }
                  frame "QAM" {
                    n141 = call "sub_qam_demod.vi"("symbol map"=w394, "symbol"=w395) -> ("bitstream"=w393:i16[])  [unwired: 9 in]
                  }
                }
                "RX Constellation Map 2" <- w383
              }
            }
            n142 = call "rx_pduExtract.vi"("output bit stream"=w374) -> ("found?"=w373:bool, "packet len"=w365:u32, "ppdu"=w372:i8[])  [unwired: 2 in]
            "found?" <- w373
            n143 = case shown="True" w373 {
              tunnel: w372 -> [_ w399]
              tunnel: w370 -> [_ w401]
              tunnel: [w396 w400] -> w369
              tunnel: w368 -> [w396 w397]
              tunnel: w365 -> [_ w398]
              frame False {
              }
              frame True {
                n144 = Enqueue Element(queue=w401, element=w399, error in (no error)=w397) -> (error out=w400:errorcluster)  [unwired: 1 in, 2 out]
                "packet len" <- w398
              }
            }
          }
        }
        n145 = global read "var_stop.vi" "system stop"() -> (w338:bool)
      }
      n146 = while {
        tunnel: w133 -> [w488]
        shift-right: [w477] -> w129
        shift-left: w132 -> [w487]
        tunnel: w128 -> [w485]
        shift-right: [w479] -> _
        shift-left: errorcluster {"status"=FALSE, "code"=0, "source"=""} ("error out") -> [w484]
        tunnel: [w478] -> w130
        i -> [w475]
        stop <- w476 stop-if-true
        # "USRP\nReceiver"
        n147 = Get Queue Status(queue=w485, error in (no error)=w484) -> (queue out=w481:refnum<queue>, error out=w480:errorcluster, # elements in queue=w483:i32)  [unwired: 1 in, 5 out]
        "# elements in queue" <- w483
        n148 = Less?(x=w483, y=5000) -> (x < y?=w473:bool)
        n149 = Greater Or Equal?(x=w475, y=25) -> (x >= y?=w472:bool)
        n150 = And(x=w473, y=w472) -> (x .and. y?=w470:bool)
        n151 = call-poly <instrlib>:"niUSRP Fetch Rx Data (poly).vi"("session handle"=w488, "number of samples"="number of samples", "error in (no error)"=w487) -> ("session handle out"=w478:refnum<k15>, "data"=w471:cluster{"t0":dbl, "dt":dbl, "Y":cdb[]}, "error out"=w477:errorcluster)  [unwired: 9 in, 1 out]
        n152 = case shown="True" w470 {
          tunnel: w481 -> [_ w493]
          tunnel: w480 -> [w489 w492]
          tunnel: [w489 w491] -> w479
          tunnel: w471 -> [_ w490]
          frame False {
          }
          frame True {
            n153 = Enqueue Element(queue=w493, element=w490, error in (no error)=w492) -> (error out=w491:errorcluster)  [unwired: 1 in, 2 out]
          }
        }
        n154 = global read "var_stop.vi" "system stop"() -> (w476:bool)
      }
      n155 = while {
        shift-right: [w503] -> w149
        shift-left: errorcluster {"status"=FALSE, "code"=0, "source"=""} ("error out") -> [w501]
        tunnel: [w502] -> w148
        tunnel: w146 -> [w500]
        tunnel: w145 -> [w498]
        shift-right: [w496] -> _
        shift-left: errorcluster {"status"=FALSE, "code"=0, "source"=""} ("error out") -> [w497]
        tunnel: w137 -> [w495]
        stop <- w494 stop-if-true
        # "USRP\nTransmitter"
        n156 = Get Queue Status(queue=w498, error in (no error)=w497) -> (queue out=w505:refnum<queue>, error out=w504:errorcluster, # elements in queue=w507:i32)  [unwired: 1 in, 5 out]
        "elements in send buffer" <- w507
        n157 = Not Equal To 0?(x=w507) -> (x != 0?=w506:bool)
        n158 = case shown="True" w506 {
          tunnel: w505 -> [_ w513]
          tunnel: w504 -> [w508 w512]
          tunnel: [w509 w511] -> w499
          tunnel: [w508 w510] -> w496
          tunnel: w495 -> [w509 _]
          frame False {
          }
          frame True {
            n159 = Dequeue Element(queue=w513, error in (no error)=w512) -> (element=w511:cluster{"t0":dbl, "dt":dbl, "Y":cdb[]}, error out=w510:errorcluster)  [unwired: 1 in, 2 out]
          }
        }
        n160 = global read "var_stop.vi" "system stop"() -> (w494:bool)
        n161 = call-poly <instrlib>:"niUSRP Write Tx Data (poly).vi"("session handle"=w500, "data"=w499, "error in (no error)"=w501) -> ("session handle out"=w502:refnum<k15>, "error out"=w503:errorcluster)  [unwired: 11 in]
      }
      n162 = call "IMAQ Dispose"("Image"=w96) -> ()  [unwired: 2 in, 4 out]
      n163 = call <instrlib>:"niUSRP Abort.vi"("session handle"=w130, "error in (no error)"=w129) -> ("session handle out"=w136:refnum<k15>, "error out"=w135:errorcluster)  [unwired: 12 in]
      n164 = call <instrlib>:"niUSRP Close Session.vi"("session handle"=w136, "error in (no error)"=w135) -> ()  [unwired: 13 in, 1 out]
      n165 = call <instrlib>:"niUSRP Close Session.vi"("session handle"=w148, "error in (no error)"=w149) -> ()  [unwired: 13 in, 1 out]
      n166 = call "IMAQ Dispose"("Image"=w97) -> ("error out"=w98:errorcluster)  [unwired: 2 in, 3 out]
      n167 = call <vilib>:"Simple Error Handler.vi"("error in (no error)"=w98) -> ()  [unwired: 1 in, 8 out]
      n168 = call <vilib>:"IMAQdx Close Camera.vi"("error in"=w85, "Session In"=w86) -> ("error out"=w89:errorcluster)  [unwired: 9 in]
      n169 = call "IMAQ Dispose"("Image"=w87, "error in (no error)"=w89) -> ("error out"=w91:errorcluster)  [unwired: 1 in, 3 out]
      n170 = Initialize Array(cdb 0.0+0.0i, 4096 ("dimension size")) -> (w111:cdb[])
      n171 = while {
        tunnel: w150 -> [w529]
        shift-right: [w526] -> _
        shift-left: errorcluster {"status"=FALSE, "code"=0, "source"=""} ("error out") -> [w532]
        tunnel: w145 -> [w525]
        shift-right: [w524] -> _
        shift-left: errorcluster {"status"=FALSE, "code"=0, "source"=""} ("error out") -> [w523]
        tunnel: w116 -> [w521]
        tunnel: w119 -> [w520]
        tunnel: w118 -> [w519]
        tunnel: w111 -> [w518]
        i -> [w517]
        stop <- w522 stop-if-true
        n172 = Greater Or Equal?(x=w517, y=100) -> (x >= y?=w514:bool)
        n173 = Get Queue Status(queue=w529, error in (no error)=w532) -> (queue out=w527:refnum<queue>, error out=w528:errorcluster, # elements in queue=w531:i32)  [unwired: 1 in, 5 out]
        n174 = Not Equal To 0?(x=w531) -> (x != 0?=w530:bool)
        n175 = And(x=w530, y=w514) -> (x .and. y?=w515:bool)
        n176 = case shown="True" w515 {
          tunnel: w528 -> [w534 w577]
          tunnel: w527 -> [_ w576]
          tunnel: [w534 w575] -> w526
          tunnel: w525 -> [_ w570]
          tunnel: [w533 w569] -> w524
          tunnel: w523 -> [w533 w568]
          tunnel: w521 -> [_ w565]
          tunnel: w520 -> [_ w564]
          tunnel: w519 -> [_ w563]
          tunnel: w518 -> [_ w553]
          frame False {
          }
          frame True {
            # "length"
            # "Waveform \nGenerator"
            n177 = Dequeue Element(queue=w576, error in (no error)=w577) -> (element=w537:i16[], error out=w575:errorcluster)  [unwired: 1 in, 2 out]
            n178 = Unbundle(w565) -> ("samples per symbol (16)"=w559:i32, "symbol map"=w552:cdb[])  [unwired: 1 out]
            n179 = Array Size(array=w537) -> (size(s)=w561:i32)
            n180 = Quotient & Remainder(x=w561, y=8) -> (floor(x/y)=w541:i32)  [unwired: 1 out]
            n181 = To Unsigned Word Integer(number=w541) -> (unsigned 16bit integer=w560:u16)
            n182 = Number To Boolean Array(number=w560) -> (Boolean array=w574:bool[])
            n183 = Reshape Array(w574, 2 ("dimension size"), 8 ("dimension size")) -> (w571:bool[][])
            n184 = for {
              tunnel: w571 -> [w580] mode=indexing
              tunnel: [w578] -> w562 mode=indexing
              n185 = Boolean Array To Number(Boolean array=w580) -> (number=w579:u32)
              n186 = To Unsigned Byte Integer(number=w579) -> (unsigned 8bit integer=w578:u8)
            }
            n187 = Initialize Array(u8 0, 128 ("dimension size")) -> (w536:u8[])
            n188 = Build Array (concatenate)(u8[] [53, 187, 37, 71, 79, 49, 4, 63] ("Array 2"), w562, w562) -> (w567:u8[])
            n189 = call "tx_pduGen.vi"("byte array"=w567) -> ("packet bits length"=→"packet bits length":i32, "pdu"=w538:i32[])  [unwired: 3 in]
            n190 = Build Array (concatenate)(w538, w537, w536) -> (w535:i32[])
            n191 = call "sub_bits_to_symbols.vi"("symbol map"=w552, "bits"=w535) -> ("symbols"=w551:cdb[])  [unwired: 9 in]
            n192 = Build Array (concatenate)(w551, w553) -> (w549:cdb[])
            n193 = call-poly <vilib>:"MT Pulse Shaping Filter.vi"("symbols"=w549, "pulse shaping filter coefficients"=w564, "samples per symbol (16)"=w559, "symbol rate (Hz)"=w563, "reset? (T)"=FALSE) -> ("output complex waveform"=w558:T9)  [unwired: 9 in, 1 out]
            n194 = Divide(x="Transmit power (db)", y=20.0) -> (x/y=w546:dbl)
            n195 = Unbundle(w558) -> ("t0"=w557:dbl, "dt"=w556:dbl, "Y"=w544:cdb[])
            n196 = Power Of 10(x=w546) -> (10^x=w545:dbl)
            n197 = Multiply(x=w544, y=w545) -> (x*y=w543:cdb[])
            n198 = Bundle(cluster=w558, "t0"=w557, "dt"=w556, "Y"=w543) -> (w555:T9)
            n199 = Enqueue Element(queue=w570, element=w555, error in (no error)=w568) -> (error out=w569:errorcluster)  [unwired: 1 in, 2 out]
          }
        }
        n200 = global read "var_stop.vi" "system stop"() -> (w522:bool)
      }
      n201 = Unbundle By Name(w91) -> ("source"=w90:string)
      n202 = call <vilib>:"Simple Error Handler.vi"("error source (\" \")"=w90, "error in (no error)"=w91) -> ("error out"=→"error out":errorcluster)  [unwired: 3 in, 4 out]
    }
    frame Error {
    }
  }
